vi "AllowUserMessages.vi"() -> ()   [LabVIEW 2016]
panel:
  out "Allow Usermessages":bool
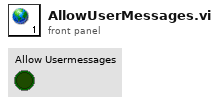
[diagram p1: front panel]
diagram:
